vi "SaveSource.vi"(8 "error in (no error)":errorcluster, 11 "VisionUI in":refnum<class "VisionUI.lvclass">) -> (0 "error out":errorcluster, 3 "VisionUI out":refnum<class "VisionUI.lvclass">)   [LabVIEW 2019, in "VisionUI.lvlib" / "VisionUI.lvclass"]
uses:
  VisionUI.lvclass
  C:/Repos/Demo/Actors/Vision/Vision/Vision.lvclass
  VisionUI.lvclass/VisionUI.ctl
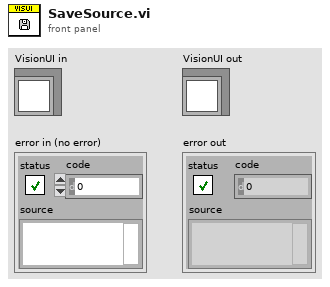
[diagram p1: front panel]
types:
  T1 = typedef "IMAQ Image.ctl" = refnum<image>
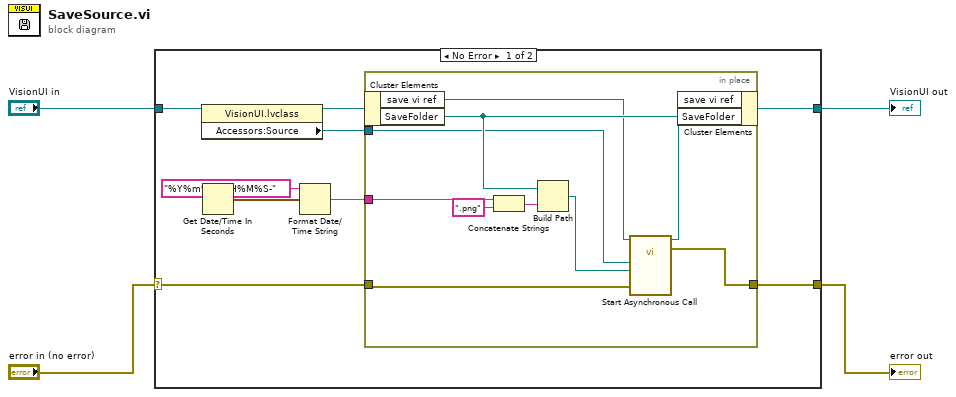
[diagram p0: block diagram]
diagram:
  n1 = case shown="No Error" "error in (no error)" {
    selector: "error in (no error)" -> [w6 w25]
    tunnel: [w5 w25] -> w1
    tunnel: [w11 w24] -> w2
    tunnel: "VisionUI in" -> [w13 w24]
    frame No Error {
      n2 = property class="VisionUI.lvclass"(reference=w13) -> (reference out=w12:refnum<class "VisionUI.lvclass">, "Accessors:Source"=w7:T1)  [unwired: 1 in, 1 out]
      n3 = Get Date/Time In Seconds() -> (seconds since 1Jan1904=w10:timestamp)
      n4 = Format Date/Time String(time format string (%c)="%Y%m%d_%H%M%S-", seconds (now)=w10) -> (date/time string=w8:string)  [unwired: 1 in]
      n5 = in-place {
        in-place-border: w8 -> [w22]
        in-place-border: w7 -> [w17]
        in-place-border: w6 -> [w15]
        in-place-border: [w14] -> w5
        n6 = in-place-cluster #1(w12) -> ("save vi ref"=w19:refnum<vi>, "SaveFolder"=w23:path)
        n7 = Concatenate Strings(w22, ".png" ("string")) -> (w21:string)
        n8 = Build Path(base path=w23, name or relative path=w21) -> (appended path=w16:path)
        n9 = call-by-ref "Start Asynchronous Call"(reference=w19, "error in (no error)"=w15, "Path"=w16, "Source"=w17) -> (reference out=w18:refnum<vi>, error out=w14:errorcluster)  [unwired: 9 in, 1 out]
        n10 = in-place-cluster #1("save vi ref"=w18, "SaveFolder"=w23) -> (w11:refnum<class "VisionUI.lvclass">)
      }
    }
    frame Error {
    }
  }
  "error out" <- w1
  "VisionUI out" <- w2
